vi "Populate Nodes List.vi"(8 "error in":errorcluster, 10 "Nodes":string[](array[string]), 11 "Home in":refnum<class "Home.lvclass">) -> (0 "error out":errorcluster, 3 "Home out":refnum<class "Home.lvclass">)   [LabVIEW 2024, in "Home.lvlib" / "Home.lvclass"]
uses:
  Home.lvclass
  Home.lvclass/Home.ctl
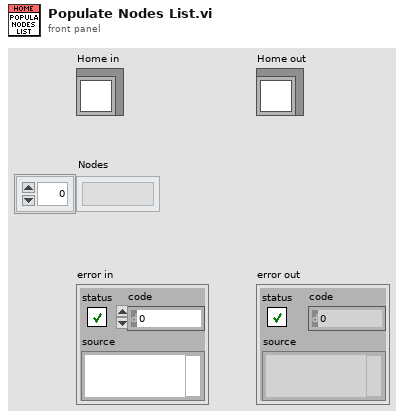
[diagram p1: front panel]
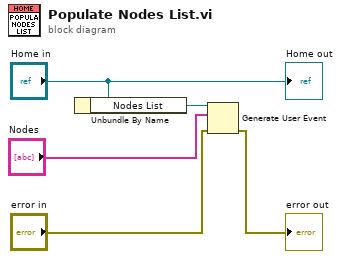
[diagram p0: block diagram]
diagram:
  n1 = Unbundle By Name("Home in") -> ("Nodes List"=w4:refnum<user-event>)
  n2 = Generate User Event(user event=w4, event data cluster="Nodes", error in="error in") -> (error out=→"error out":errorcluster)  [unwired: 1 in, 1 out]
  "Home out" <- "Home in"
